vi "UI_Hide.vi"(8 "error in (no error)":errorcluster, 11 "UI_Actor in":refnum<class "UI_Actor.lvclass">) -> (0 "error out":errorcluster, 3 "UI_Actor out":refnum<class "UI_Actor.lvclass">)   [LabVIEW 2020, in "UI_Actor.lvlib" / "UI_Actor.lvclass"]
uses:
  UI_Actor.lvclass
  UI_Actor.lvclass/UI_Actor.ctl
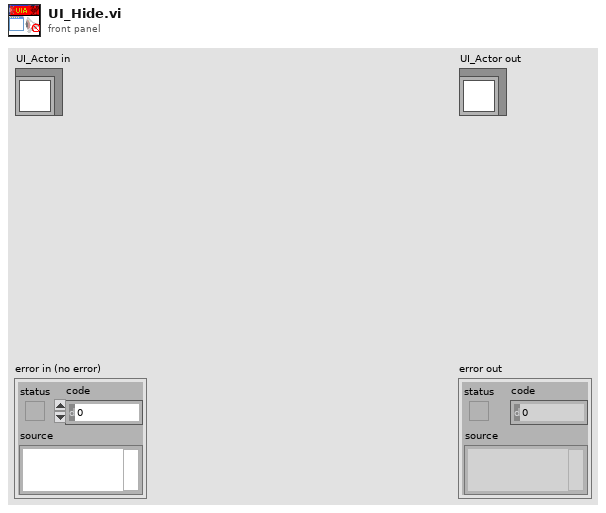
[diagram p1: front panel]
types:
  T1 = enum32{"Invalid", "Standard", "Closed", "Hidden", "Minimized", "Maximized"}
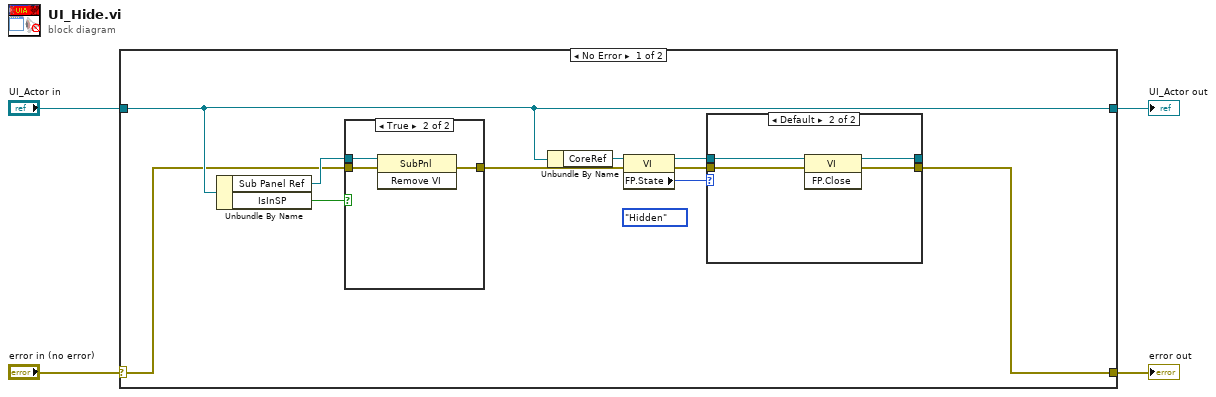
[diagram p0: block diagram]
diagram:
  n1 = case shown="No Error" "error in (no error)" {
    selector: "error in (no error)" -> [w6 w26]
    tunnel: [w10 w26] -> w1
    tunnel: [w7 w25] -> w3
    tunnel: "UI_Actor in" -> [w7 w25]
    frame No Error {
      (unwired) T1."Hidden" ("y")
      n2 = Unbundle By Name(w7) -> ("Sub Panel Ref"=w8:refnum<vi>, "IsInSP"=w9:bool)
      n3 = case shown="True" w9 {
        tunnel: w6 -> [w15 w18]
        tunnel: w8 -> [_ w17]
        tunnel: [w15 w16] -> w5
        frame False {
        }
        frame True {
          n4 = invoke on="Invoke Node" class="SubPnl" method="Remove VI"(reference=w17, error in=w18) -> (error out=w16:errorcluster)  [unwired: 1 in, 2 out]
        }
      }
      n5 = Unbundle By Name(w7) -> ("CoreRef"=w12:refnum<vi>)
      n6 = property class="VI"(reference=w12, error in=w5) -> (reference out=w13:refnum<vi>, error out=w11:errorcluster, "FP.State"=w14:T1)
      n7 = case shown="Default" w14 {
        tunnel: [w20 w23] -> _
        tunnel: w13 -> [w20 w24]
        tunnel: w11 -> [w19 w21]
        tunnel: [w19 w22] -> w10
        frame "Invalid", "Closed" {
        }
        frame Default {
          n8 = invoke class="VI" method="FP.Close"(reference=w24, error in=w21) -> (reference out=w23:refnum<vi>, error out=w22:errorcluster)  [unwired: 1 in, 1 out]
        }
      }
    }
    frame Error {
    }
  }
  "error out" <- w1
  "UI_Actor out" <- w3
